vi "findSetParamsHelper.vi"(0 "params in":refnum<class "JSON Value.lvclass">, 1 "inputDataDictionary":refnum<class "data dictionary.lvclass">, 11 "error in":errorcluster) -> (3 "tagindex":i32, 4 "params out":refnum<class "JSON Value.lvclass">, 6 "tagname":string, 8 "tagtype":T2, 10 "tagdata":T1, 13 "invalidTagType":string, 14 "missingParam":string, 15 "error out":errorcluster)   [LabVIEW 2017, in "JSON_RPC_Interface runtime.lvclass"]
uses:
  JSON_RPC_Interface runtime.lvclass
  <vilib>/NI/JSON Support for LabVIEW/JSON Value/JSON Value.lvclass
  <vilib>/NI/Tag Bus/tag/Data Type.ctl
  <vilib>/NI/Tag Bus/dictionary/data dictionary.lvclass
  <vilib>/NI/JSON Support for LabVIEW/JSON Value/Read Value/Read value (String).vi
  <vilib>/NI/JSON Support for LabVIEW/JSON Value/Read Value/Read value (Numeric).vi
  <vilib>/NI/JSON Support for LabVIEW/JSON Value/Read Value/Read value (Boolean).vi
  <vilib>/NI/JSON Support for LabVIEW/JSON Value/Array/Get Array Values/Get Array Values (Numeric[]).vi
  <vilib>/NI/JSON Support for LabVIEW/JSON Value/Array/Get Array Values/Get Array Values (Boolean[]).vi
  <vilib>/NI/JSON Support for LabVIEW/JSON Value/Array/Get Array Values/Get Array Values (String[]).vi
  <vilib>/NI/Tag Bus/tag/tag descriptor.lvclass
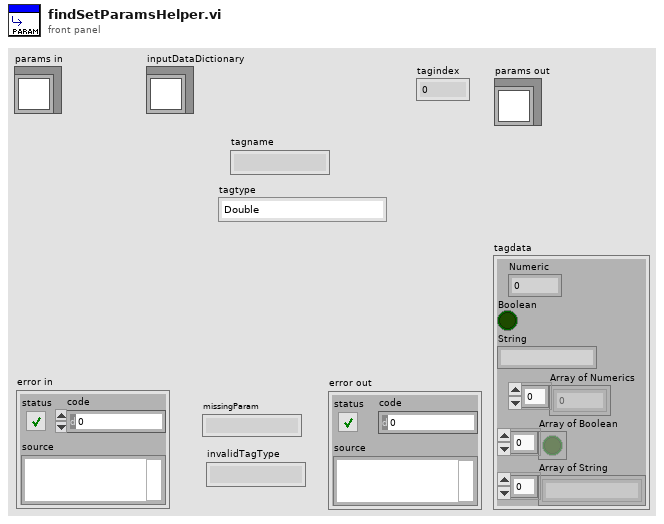
[diagram p1: front panel]
types:
  T1 = cluster{"Numeric":dbl, "Boolean":bool, "String":string, "Array of Numerics":dbl[], "Array of Boolean":bool[], "Array of String":string[]}
  T2 = typedef "tag bus.lvlib/tag descriptor.lvclass/Data Type.ctl" = enum16{"Double", "Single", "I64", "I32", "I16", "I8", "U64", "U32", "U16", "U8", "Boolean", "String", "Array of Double", "Array of Single", "Array of I64", "Array of I32", "Array of I16", "Array of I8", "Array of U64", "Array of U32", "Array of U16", "Array of U8", "Array of Boolean", "Array of String"}
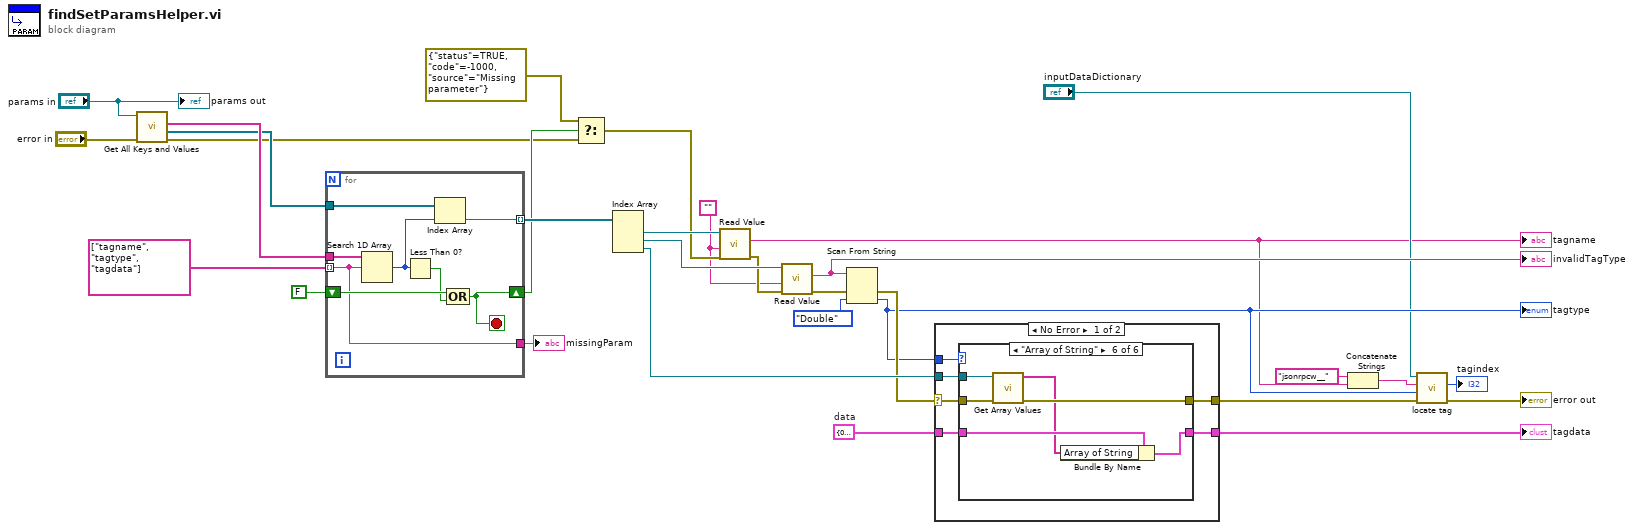
[diagram p0: block diagram]
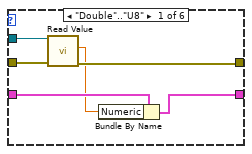
[diagram p2: hidden frame]
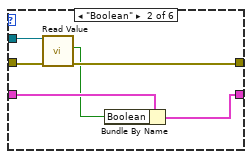
[diagram p3: hidden frame]
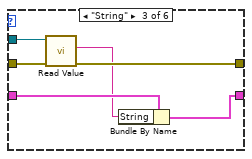
[diagram p4: hidden frame]
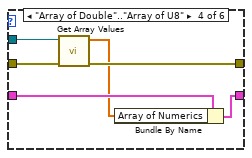
[diagram p5: hidden frame]
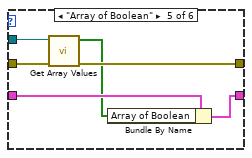
[diagram p6: hidden frame]
diagram:
  w10 = T1 {"Numeric"=0.0, "Boolean"=FALSE, "String"="", "Array of Numerics"=[], "Array of Boolean"=[], "Array of String"=[]}  # data
  w16 = ""
  n1 = call <vilib>:"Get All Keys and Values.vi"("error in"="error in", "JSON Value in"="params in") -> ("error out"=w20:errorcluster, "values"=w25:refnum<class "JSON Value.lvclass">[], "keys"=w30:string[])  [unwired: 7 in]
  n2 = for {
    tunnel: w30 -> [w39]
    tunnel: w25 -> [w34]
    tunnel: string[] ["tagname", "tagtype", "tagdata"] -> [w35] mode=indexing
    shift-right: [w36] -> w21
    shift-left: FALSE -> [w38]
    tunnel: [w35] -> w17
    tunnel: [w32] -> w22 mode=indexing
    stop <- w36 stop-if-true
    n3 = Search 1D Array(1D array=w39, element=w35) -> (index of element=w33:i32)  [unwired: 1 in]
    n4 = Less Than 0?(x=w33) -> (x < 0?=w37:bool)
    n5 = Index Array(array=w34, index=w33) -> (element=w32:refnum<class "JSON Value.lvclass">)
    n6 = Compound Arithmetic op=OR(w38, w37) -> (w36:bool)
  }
  "missingParam" <- w17
  n7 = Select(t=errorcluster {"status"=TRUE, "code"=-1000, "source"="Missing parameter"}, s=w21, f=w20) -> (s? t:f=w19:errorcluster)
  n8 = Index Array(array=w22) -> (element #1=w28:refnum<class "JSON Value.lvclass">, element #2=w27:refnum<class "JSON Value.lvclass">, element #3=w12:refnum<class "JSON Value.lvclass">)  [unwired: 3 in]
  n9 = call-poly <vilib>:"Read Value.vi"("error in (no error)"=w19, "default value"=w16, "JSON String in"=w28) -> ("error out"=w26:errorcluster, "value"=w3:string)  [unwired: 6 in, 1 out]
  "tagname" <- w3
  n10 = call-poly <vilib>:"Read Value.vi"("error in (no error)"=w26, "default value"=w16, "JSON String in"=w27) -> ("error out"=w14:errorcluster, "value"=w13:string)  [unwired: 6 in, 1 out]
  "invalidTagType" <- w13
  n11 = Scan From String(input string=w13, error in=w14, default 1=Data_Type."Double" ("Data Type")) -> (error out=w11:errorcluster, output 1=w7:T2)  [unwired: 2 in, 2 out]
  "tagtype" <- w7
  n12 = case shown="No Error" w11 {
    selector: w11 -> [w42 w83]
    tunnel: w12 -> [w45 _]
    tunnel: [w44 w83] -> w8
    tunnel: w7 -> [w43 _]
    tunnel: w10 -> [w41 w82]
    tunnel: [w40 w82] -> w9
    frame No Error {
      n13 = case shown="\"Array of String\"" w43 {
        tunnel: w45 -> [w51 w57 w61 w69 w75 w81]
        tunnel: [w49 w55 w62 w67 w73 w79] -> w44
        tunnel: w42 -> [w50 w56 w63 w68 w74 w80]
        tunnel: w41 -> [w48 w54 w60 w66 w72 w78]
        tunnel: [w46 w52 w58 w64 w70 w76] -> w40
        frame "Double".."U8" {
          n14 = call-poly <vilib>:"Read Value.vi"("error in (no error)"=w50, "JSON Numeric in"=w51) -> ("error out"=w49:errorcluster, "value"=w47:dbl)  [unwired: 7 in, 1 out]
          n15 = Bundle By Name(cluster=w48, "Numeric"=w47) -> (w46:T1)
        }
        frame "Boolean" {
          n16 = call-poly <vilib>:"Read Value.vi"("error in (no error)"=w56, "JSON Boolean in"=w57) -> ("error out"=w55:errorcluster, "value"=w53:bool)  [unwired: 7 in, 1 out]
          n17 = Bundle By Name(cluster=w54, "Boolean"=w53) -> (w52:T1)
        }
        frame "String" {
          n18 = call-poly <vilib>:"Read Value.vi"("error in (no error)"=w63, "JSON String in"=w61) -> ("error out"=w62:errorcluster, "value"=w59:string)  [unwired: 7 in, 1 out]
          n19 = Bundle By Name(cluster=w60, "String"=w59) -> (w58:T1)
        }
        frame "Array of Double".."Array of U8" {
          n20 = call-poly <vilib>:"Get Array Values.vi"("error in (no error)"=w68, "JSON Value in"=w69) -> ("error out"=w67:errorcluster, "values"=w65:dbl[])  [unwired: 8 in]
          n21 = Bundle By Name(cluster=w66, "Array of Numerics"=w65) -> (w64:T1)
        }
        frame "Array of Boolean" {
          n22 = call-poly <vilib>:"Get Array Values.vi"("error in (no error)"=w74, "JSON Value in"=w75) -> ("error out"=w73:errorcluster, "values"=w71:bool[])  [unwired: 8 in]
          n23 = Bundle By Name(cluster=w72, "Array of Boolean"=w71) -> (w70:T1)
        }
        frame "Array of String" {
          n24 = call-poly <vilib>:"Get Array Values.vi"("error in (no error)"=w80, "JSON Value in"=w81) -> ("error out"=w79:errorcluster, "values"=w77:string[])  [unwired: 8 in]
          n25 = Bundle By Name(cluster=w78, "Array of String"=w77) -> (w76:T1)
        }
      }
    }
    frame Error {
    }
  }
  "tagdata" <- w9
  n26 = Concatenate Strings("jsonrpcw__" ("string"), w3) -> (w2:string)
  n27 = call <vilib>:"locate tag.vi"("error in"=w8, "data type"=w7, "name"=w2, "data dictionary in"="inputDataDictionary") -> ("error out"=→"error out":errorcluster, "index"=→"tagindex":i32)  [unwired: 5 in, 1 out]
  "params out" <- "params in"
